vi "BeepGen.vi"(7 "Numeric in":dbl, 10 "Wait time before beep":dbl, 11 "Time b/w Beeps (ms)":dbl) -> (2 "In Range?":bool, 3 "Numeric out":dbl)   [LabVIEW 2020]
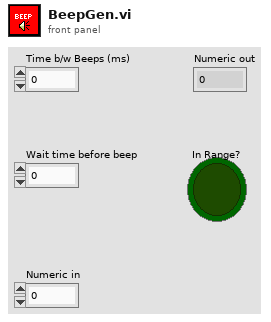
[diagram p1: front panel]
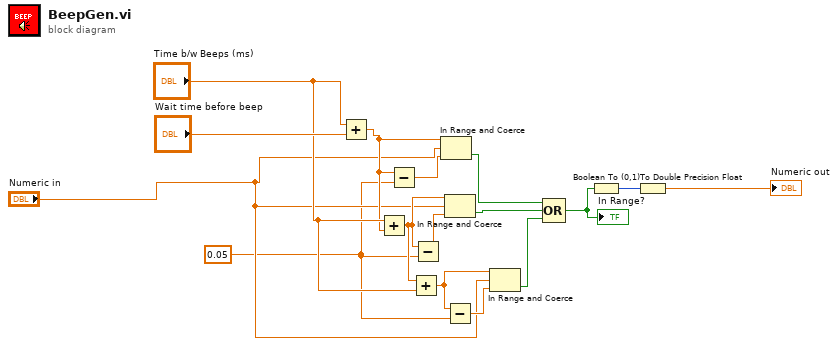
[diagram p0: block diagram]
diagram:
  w1 = 0.05
  n1 = Add(x="Time b/w Beeps (ms)", y="Wait time before beep") -> (x+y=w4:dbl)
  n2 = Add(x="Time b/w Beeps (ms)", y=w4) -> (x+y=w8:dbl)
  n3 = Subtract(x=w4, y=w1) -> (x-y=w3:dbl)
  n4 = Add(x=w8, y="Time b/w Beeps (ms)") -> (x+y=w9:dbl)
  n5 = Subtract(x=w8, y=w1) -> (x-y=w5:dbl)
  n6 = In Range and Coerce(upper limit=w4, x="Numeric in", lower limit=w3) -> (In Range?=w6:bool)  [unwired: 1 out]
  n7 = In Range and Coerce(upper limit=w8, x="Numeric in", lower limit=w5) -> (In Range?=w7:bool)  [unwired: 1 out]
  n8 = Subtract(x=w9, y=w1) -> (x-y=w10:dbl)
  n9 = In Range and Coerce(upper limit=w9, x="Numeric in", lower limit=w10) -> (In Range?=w11:bool)  [unwired: 1 out]
  n10 = Compound Arithmetic op=OR(w6, w7, w11) -> (w12:bool)
  "In Range?" <- w12
  n11 = Boolean To (0,1)(Boolean=w12) -> (0, 1=w13:i16)
  n12 = To Double Precision Float(number=w13) -> (double precision float=→"Numeric out":dbl)
